vi "DetermineRF name.vi"(7 "Inst:Test Name":string, 10 "Complex FRF":cluster{"t0":dbl, "dt":dbl, "Y":cdb[]}, 11 "Last Path":path) -> (2 "Y":cdb[](array[numeric]), 3 "Header Info":T1, 4 "trf file":path, 5 "Path to csv Folder":path)   [LabVIEW 2022 SP3]
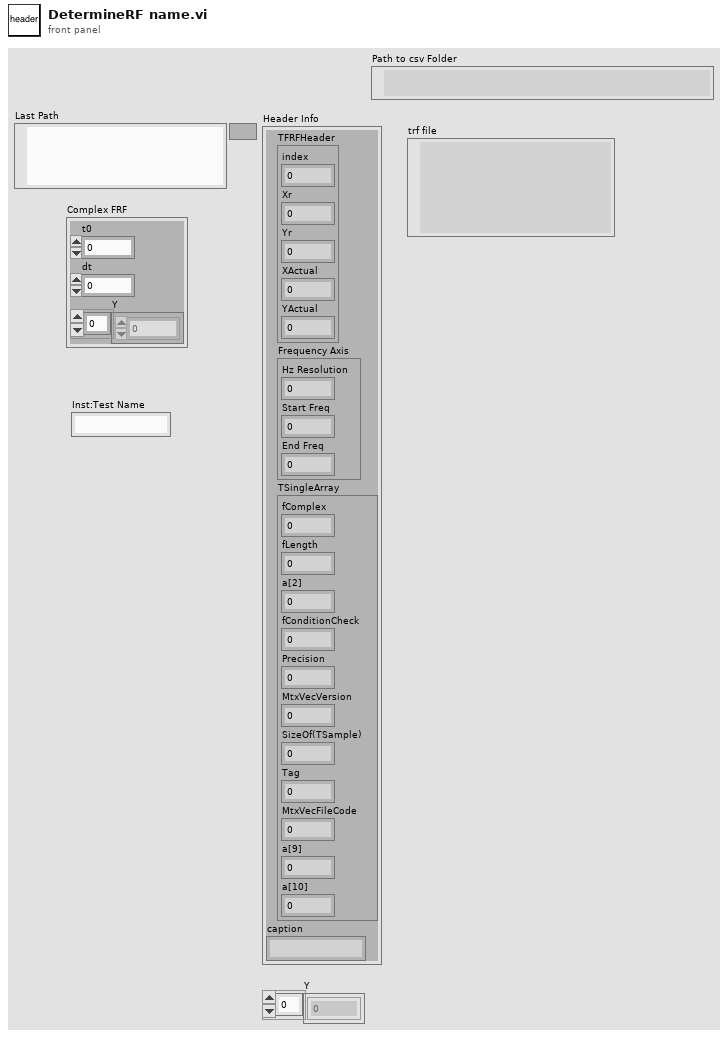
[diagram p1: front panel]
types:
  T1 = cluster{"TFRFHeader":cluster{"index":u32, "Xr":dbl, "Yr":dbl, "XActual":dbl, "YActual":dbl}, "Frequency Axis":cluster{"Hz Resolution":dbl, "Start Freq":dbl, "End Freq":dbl}, "TSingleArray":cluster{"fComplex":u32, "fLength":dbl, "a[2]":dbl, "fConditionCheck":dbl, "Precision":dbl, "MtxVecVersion":dbl, "SizeOf(TSample)":dbl, "Tag":dbl, "MtxVecFileCode":dbl, "a[9]":dbl, "a[10]":dbl}, "caption":string}
  T2 = cluster{"Test":string, "Set":string, "Position":string, "Tap":string}
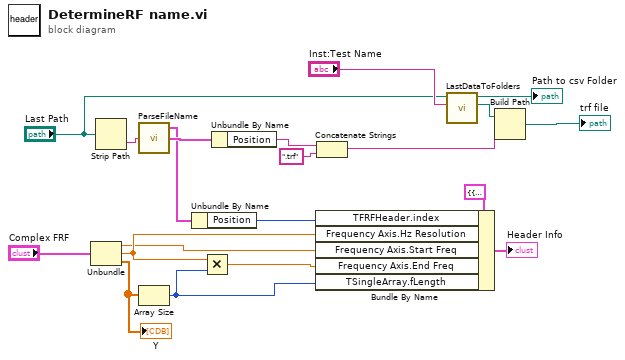
[diagram p0: block diagram]
diagram:
  n1 = Unbundle("Complex FRF") -> ("t0"=w15:dbl, "dt"=w18:dbl, "Y"=w16:cdb[])
  "Y" <- w16
  n2 = Strip Path(path="Last Path") -> (name=w12:string)  [unwired: 1 out]
  n3 = call "ParseFileName.vi"("String in"=w12) -> ("Info"=w14:cluster{"Set":string, "Position":i32, "Tap":i32}, "Name"=w20:T2)  [unwired: 1 out]
  n4 = Array Size(array=w16) -> (size(s)=w17:i32)
  n5 = Unbundle By Name(w14) -> ("Position"=w13:i32)
  n6 = Multiply(x=w18, y=w17) -> (x*y=w19:dbl)
  n7 = Unbundle By Name(w20) -> ("Position"=w8:string)
  n8 = Bundle By Name(cluster=T1 {"TFRFHeader"={"index"=11, "Xr"=0.0, "Yr"=0.0, "XActual"=0.0, "YActual"=0.0}, "Frequency Axis"={"Hz Resolution"=0.732421875, "Start Freq"=199.951171875, "End Freq"=9999.755859375}, "TSingleArray"={"fComplex"=1, "fLength"=13381.0, "a[2]"=0.0, "fConditionCheck"=1.0, "Precision"=0.0, "MtxVecVersion"=420.0, "SizeOf(TSample)"=8.0, "Tag"=0.0, "MtxVecFileCode"=64019.0, "a[9]"=0.0, "a[10]"=0.0}, "caption"="\u0000\u0000\u0000\u0000"} ("Header Info"), "TFRFHeader.index"=w13, "Frequency Axis.Hz Resolution"=w18, "Frequency Axis.Start Freq"=w15, "Frequency Axis.End Freq"=w19, "TSingleArray.fLength"=w17) -> (→"Header Info":T1)
  n9 = Concatenate Strings(w8, ".trf" ("string")) -> (w7:string)
  n10 = call "LastDataToFolders.vi"("Inst:Test Name"="Inst:Test Name", "Last Path"="Last Path") -> ("Path To TRF Folder"=w3:path, "Path to csv Folder"=→"Path to csv Folder":path)  [unwired: 7 in, 1 out]
  n11 = Build Path(base path=w3, name or relative path=w7) -> (appended path=→"trf file":path)
